vi "LocalVariable.vi"() -> ()   [LabVIEW 2019]
panel:
  out "x*y":dbl
  out "Numeric 2":dbl
  in  "Numeric":dbl
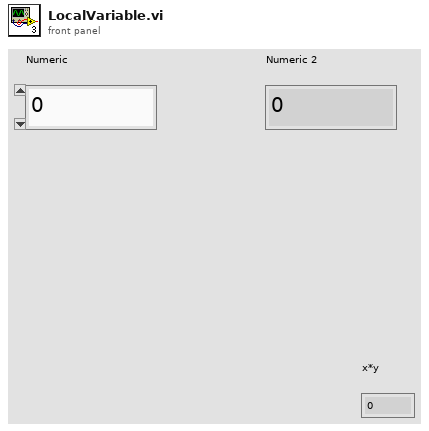
[diagram p1: front panel]
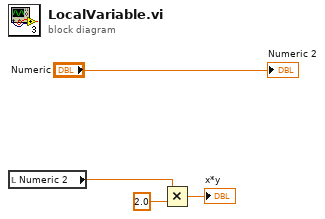
[diagram p0: block diagram]
diagram:
  n1 = local read "Numeric 2"() -> (w3:dbl)
  n2 = Multiply(x=w3, y=2.0) -> (x*y=→"x*y":dbl)
  "Numeric 2" <- "Numeric"
